vi "LoadCellReadings.vi"(6 "Arduino Load Cell Readings?":refnum<visa-resource-name>) -> (7 "read buffer":string)   [LabVIEW 2023]
uses:
  <vilib>/Instr/_visa.llb/VISA Configure Serial Port (Instr).vi
  <vilib>/Utility/file.llb/Write Delimited Spreadsheet (string).vi
panel:
  in  "stop":bool
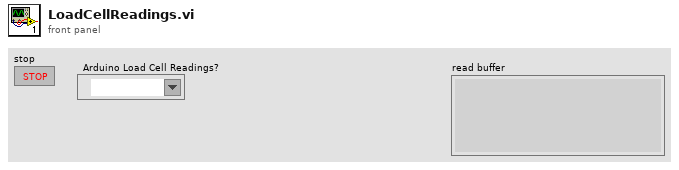
[diagram p1: front panel]
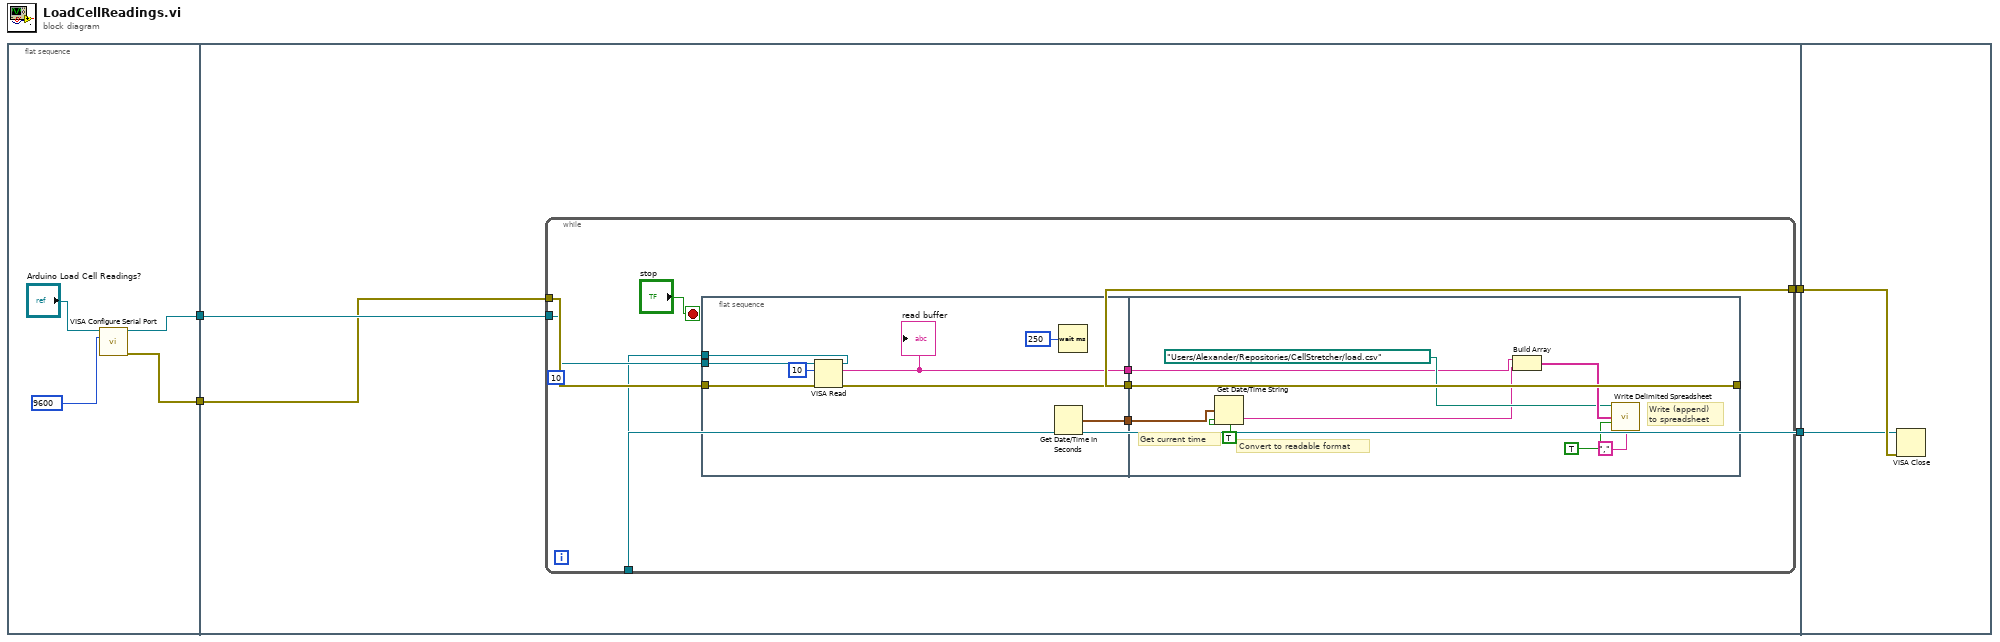
[diagram p0: block diagram]
diagram:
  n1 = flat-sequence {
    tunnel: [w7] -> w2
    tunnel: [w6] -> w1
    tunnel: [w12] -> w4
    tunnel: [w11] -> w3
    tunnel: w2 -> [w10]
    tunnel: w1 -> [w9]
    tunnel: w4 -> [w39]
    tunnel: w3 -> [w38]
    frame #0 {
      n2 = call-poly "VISA Configure Serial Port"("VISA resource name"="Arduino Load Cell Readings?", "baud rate (9600)"=u32 9600) -> ("VISA resource name out"=w7:refnum<visa-resource-name>, "error out"=w6:errorcluster)  [unwired: 12 in]
    }
    frame #1 {
      (unwired) u32 10 ("byte count")
      n3 = while {
        tunnel: [w17] -> w12
        tunnel: [w16] -> w11
        tunnel: w10 -> [w18]
        tunnel: w9 -> [w19]
        stop <- "stop" stop-if-true
        n4 = flat-sequence {
          tunnel: w19 -> [w28]
          tunnel: w18 -> [w26]
          tunnel: [w24] -> w16
          tunnel: [w25] -> w15
          tunnel: [w23] -> w14
          tunnel: [w21] -> w13
          tunnel: [w37] -> w17
          tunnel: w15 -> [w37]
          tunnel: w14 -> [w30]
          tunnel: w13 -> [w29]
          frame #0 {
            n5 = VISA Read(VISA resource name=w26, byte count=u32 10, error in (no error)=w28) -> (VISA resource name out=w24:refnum<visa-resource-name>, read buffer=w23:string, error out=w25:errorcluster)  [unwired: 1 out]
            "read buffer" <- w23
            n6 = Get Date/Time In Seconds() -> (seconds since 1Jan1904=w21:timestamp)
            n7 = Wait (ms)(milliseconds to wait=u32 250) -> ()  [unwired: 1 out]
          }
          frame #1 {
            # "Get current time"
            # "Convert to readable format"
            # "Write (append) to spreadsheet"
            n8 = Get Date/Time String(seconds (now)=w29, want seconds? (F)=TRUE) -> (time string=w31:string)  [unwired: 1 in, 1 out]
            n9 = Build Array(w30, w31) -> (w36:string[])
            n10 = call-poly <vilib>:"Write Delimited Spreadsheet.vi"("file path (dialog if empty)"=path "/Users/Alexander/Repositories/CellStretcher/load.csv", "1D data"=w36, "append to file? (new file:F)"=TRUE, "delimiter (\\t)"="," ("delimiter (\\t)")) -> ()  [unwired: 10 in, 2 out]
          }
        }
      }
    }
    frame #2 {
      n11 = VISA Close(VISA resource name=w38, error in (no error)=w39) -> ()  [unwired: 1 out]
    }
  }
